vi "Extract Channel List.vi"(0 "config file path":path=path "C:/Documents and Settings/Jenkins/My Documents/Projects/W03247 Delphi DAQ Cart/CODE/System/system.ini", 5 "channel group":T3(ring), 11 "error in (no error)":errorcluster) -> (4 "config file path (dup)":path, 6 "App Channels":T1, 15 "error out":errorcluster)   [LabVIEW 2019]
uses:
  Type Defs and Controls/Channel Cluster.ctl
  Type Defs and Controls/Channel Config.ctl
  <vilib>/Utility/config.llb/Read Key (String).vi
  <vilib>/Utility/config.llb/NI_LVConfig.lvlib
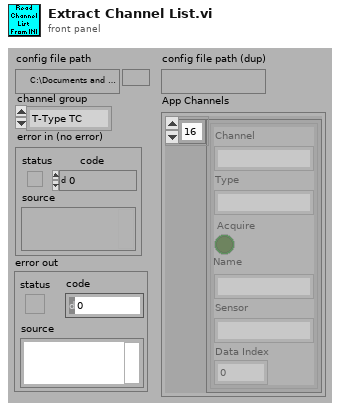
[diagram p1: front panel]
types:
  T1 = typedef "Channel Cluster.ctl" = cluster{"Channels":T2[]}
  T2 = typedef "Channel Config.ctl" = cluster{"Channel":string, "Type":string, "Acquire":bool, "Name":string, "Sensor":string, "Data Index":u32}
  T3 = enum16{"T-Type TC", "T-Type TC #2", "AI", "AI #2"}
  T4 = typedef "NI_LVConfig.lvlib/Config Data RefNum.ctl" = refnum<k1>
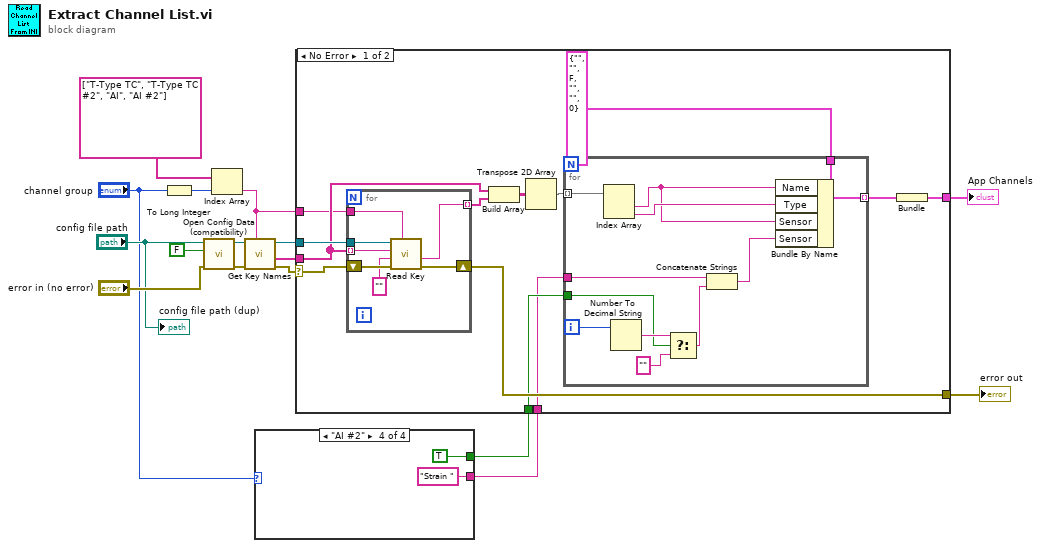
[diagram p0: block diagram]
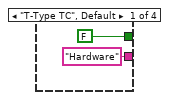
[diagram p2: hidden frame]
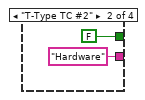
[diagram p3: hidden frame]
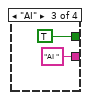
[diagram p4: hidden frame]
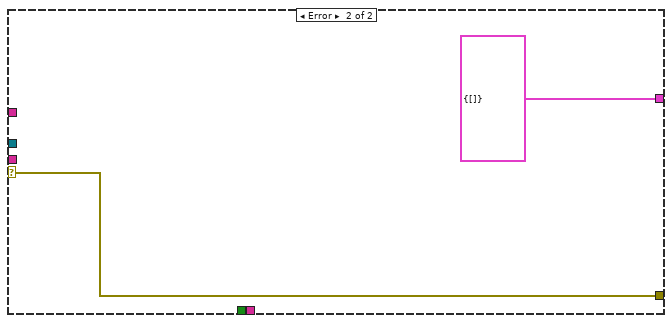
[diagram p5: hidden frame]
diagram:
  n1 = To Long Integer(number="channel group") -> (32bit integer=w9:i32)
  n2 = call <vilib>:"Open Config Data (compatibility).vi"("error in (no error)"="error in (no error)", "create file if necessary (T)"=FALSE ("create file if necessary? (T)"), "configuration file path"="config file path") -> ("error out"=w14:errorcluster, "refnum"=w15:T4)  [unwired: 6 in, 1 out]
  n3 = Index Array(array=string[] ["T-Type TC", "T-Type TC #2", "AI", "AI #2"], index=w9) -> (element=w10:string)
  n4 = call <vilib>:"Get Key Names.vi"("section"=w10, "error in (no error)"=w14, "refnum"=w15) -> ("error out"=w7:errorcluster, "key names"=w12:string[], "refnum out"=w13:T4)  [unwired: 5 in, 1 out]
  n5 = case shown="\"AI #2\"" "channel group" {
    tunnel: ["Hardware" "Hardware" "AI " "Strain "] -> w1
    tunnel: [FALSE FALSE TRUE TRUE] -> w2
    frame "T-Type TC", Default {
    }
    frame "T-Type TC #2" {
    }
    frame "AI" {
    }
    frame "AI #2" {
    }
  }
  n6 = case shown="No Error" w7 {
    selector: w7 -> [w32 w58]
    tunnel: w13 -> [w37 _]
    tunnel: w12 -> [w35 _]
    tunnel: w10 -> [w33 _]
    tunnel: [w31 w58] -> w6
    tunnel: [w28 cluster{T2[]} {[]}] -> w4
    tunnel: w2 -> [w26 _]
    tunnel: w1 -> [w25 _]
    frame No Error {
      n7 = for {
        tunnel: w37 -> [w56]
        tunnel: w33 -> [w55]
        tunnel: w35 -> [w54] mode=indexing
        shift-right: [w52] -> w31
        shift-left: w32 -> [w53]
        tunnel: [w50] -> w36 mode=indexing
        n8 = call-poly <vilib>:"Read Key.vi"("section"=w55, "error in (no error)"=w53, "default value"="", "key"=w54, "refnum"=w56) -> ("error out"=w52:errorcluster, "value"=w50:string)  [unwired: 3 in, 2 out]
      }
      n9 = Build Array(w35, w36) -> (w34:string[][])
      n10 = Transpose 2D Array(2D array=w34) -> (transposed array=w30:string[][])
      n11 = for {
        tunnel: w30 -> [w49] mode=indexing
        tunnel: T2 {"Channel"="", "Type"="", "Acquire"=FALSE, "Name"="", "Sensor"="", "Data Index"=0} ("Channel") -> [w48]
        tunnel: [w46] -> w29 mode=indexing
        tunnel: w26 -> [w42]
        tunnel: w25 -> [w40]
        i -> [w38]
        n12 = Index Array(array=w49) -> (element #1=w45:string, element #2=w47:string)  [unwired: 2 in]
        n13 = Number To Decimal String(number=w38) -> (decimal integer string=w44:string)  [unwired: 1 in]
        n14 = Select(t=w44, s=w42, f="") -> (s? t:f=w41:string)
        n15 = Concatenate Strings(w40, w41) -> (w39:string)
        n16 = Bundle By Name(cluster=w48, "Name"=w45, "Type"=w47, "Sensor"=w45, "Sensor"=w39) -> (w46:T2)
      }
      n17 = Bundle(w29) -> (w28:cluster{T2[]})  [unwired: 1 in]
    }
    frame Error {
    }
  }
  "error out" <- w6
  "App Channels" <- w4
  "config file path (dup)" <- "config file path"
